vi "Init.vi"(8 "error in":errorcluster, 11 "VISA resource in":refnum<visa-resource-name>) -> (0 "error out":errorcluster, 1 "Passed Init?":bool, 2 "Instrument IDN":string, 3 "VISA resource out":refnum<visa-resource-name>)   [LabVIEW 2025]
uses:
  <vilib>/Utility/error.llb/Trim Whitespace One-Sided.vi
  <vilib>/Instr/_visa.llb/VISA Configure Serial Port (Instr).vi
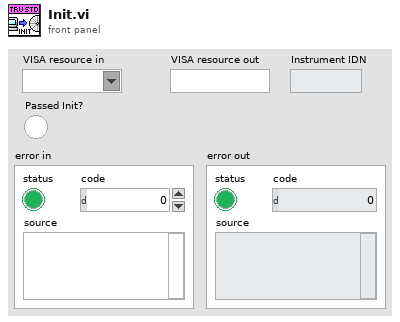
[diagram p1: front panel]
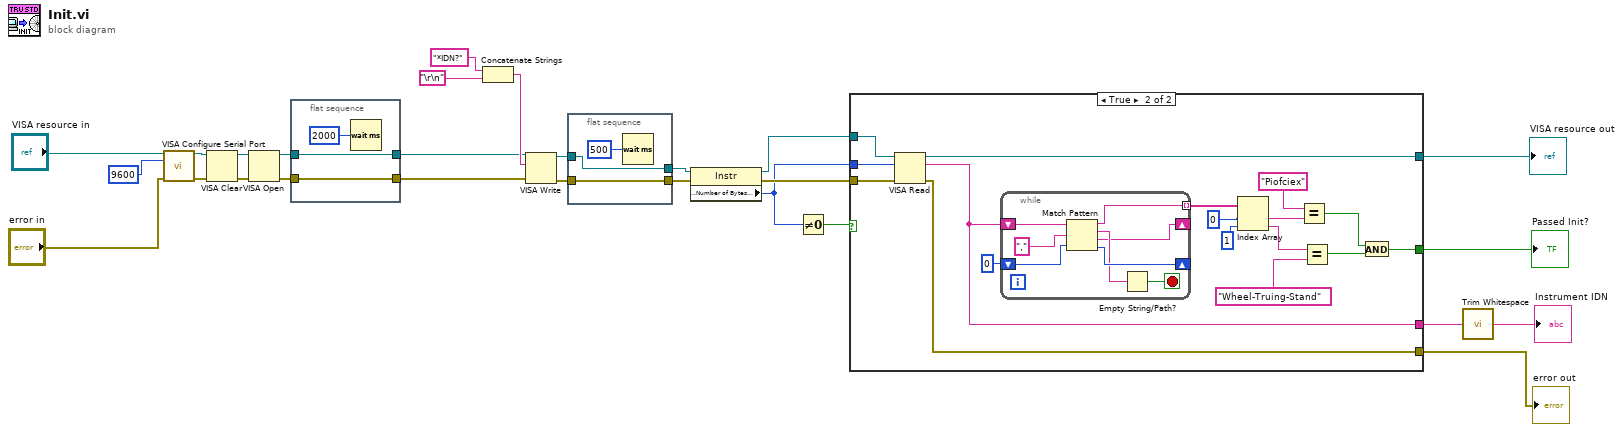
[diagram p0: block diagram]
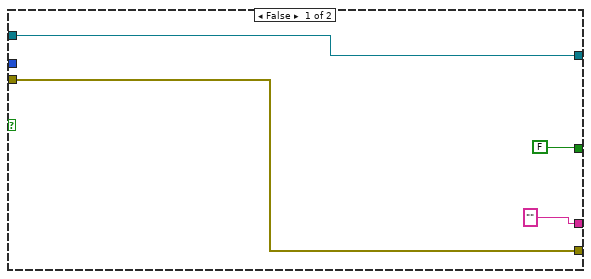
[diagram p2: hidden frame]
diagram:
  n1 = call-poly "VISA Configure Serial Port"("VISA resource name"="VISA resource in", "baud rate (9600)"=u32 9600, "error in (no error)"="error in") -> ("VISA resource name out"=w8:refnum<visa-resource-name>, "error out"=w11:errorcluster)  [unwired: 11 in]
  n2 = VISA Clear(VISA resource name=w8, error in (no error)=w11) -> (VISA resource name out=w9:refnum<visa-resource-name>, error out=w10:errorcluster)
  n3 = VISA Open(error in (no error)=w10, VISA resource name=w9) -> (VISA resource name=w13:refnum<visa-resource-name>, error out=w12:errorcluster)  [unwired: 3 in]
  n4 = flat-sequence {
    tunnel: [w29] -> w7
    tunnel: w13 -> [w29]
    tunnel: [w28] -> w6
    tunnel: w12 -> [w28]
    frame #0 {
      n5 = Wait (ms)(milliseconds to wait=u32 2000) -> ()  [unwired: 1 out]
    }
  }
  n6 = Concatenate Strings("*IDN?" ("string"), "\r\n") -> (w26:string)
  n7 = VISA Write(VISA resource name=w7, write buffer=w26, error in (no error)=w6) -> (VISA resource name out=w19:refnum<visa-resource-name>, error out=w22:errorcluster)  [unwired: 1 out]
  n8 = flat-sequence {
    tunnel: [w32] -> w20
    tunnel: w19 -> [w32]
    tunnel: [w31] -> w21
    tunnel: w22 -> [w31]
    frame #0 {
      n9 = Wait (ms)(milliseconds to wait=u32 500) -> ()  [unwired: 1 out]
    }
  }
  n10 = property class="Instr"(reference=w20, error in=w21) -> (reference out=w24:refnum<visa-resource-name>, error out=w23:errorcluster, "Serial Settings:Number of Bytes at Serial Port"=w15:u32)
  n11 = Not Equal To 0?(x=w15) -> (x != 0?=w16:bool)
  n12 = case shown="True" w16 {
    tunnel: w15 -> [_ w54]
    tunnel: w24 -> [w37 w53]
    tunnel: w23 -> [w35 w52]
    tunnel: [w37 w48] -> w18
    tunnel: [FALSE w40] -> w17
    tunnel: [w35 w39] -> w14
    tunnel: ["" ("read buffer") w38] -> w2
    frame False {
    }
    frame True {
      n13 = VISA Read(VISA resource name=w53, byte count=w54, error in (no error)=w52) -> (VISA resource name out=w48:refnum<visa-resource-name>, read buffer=w38:string, error out=w39:errorcluster)  [unwired: 1 out]
      n14 = while {
        shift-right: [w59] -> _
        shift-left: 0 -> [w60]
        shift-right: [w56] -> _
        shift-left: w38 -> [w62]
        tunnel: [w55] -> w50 mode=indexing
        stop <- w58 stop-if-true
        n15 = Match Pattern(string=w62, regular expression="," ("search string/char (-)"), offset (0)=w60) -> (before substring=w55:string, match substring=w57:string, after substring=w56:string, offset past match=w59:i32)
        n16 = Empty String/Path?(string/path=w57) -> (empty?=w58:bool)
      }
      n17 = Index Array(array=w50, index #1=0 ("index"), index #2=1 ("index")) -> (element #1=w44:string, element #2=w45:string)
      n18 = Equal?(x="Piofciex", y=w44) -> (x = y?=w42:bool)
      n19 = Equal?(x=w45, y="Wheel-Truing-Stand") -> (x = y?=w41:bool)
      n20 = And(x=w42, y=w41) -> (x .and. y?=w40:bool)
    }
  }
  "VISA resource out" <- w18
  "Passed Init?" <- w17
  "error out" <- w14
  n21 = call <vilib>:"Trim Whitespace.vi"("string"=w2) -> ("trimmed string"=→"Instrument IDN":string)  [unwired: 1 in]
